vi "_Update TIC Property.vi"(10 "Current Data":T2={"Scan#"=0, "Run Time (mS)"=0, "TIC X"=[], "TIC Y"=[], "MassRange"=[], "Fixed Mass (amu)"=1.0, "Method"={"StartT(mS)"=0, "#Cycles"=0, "PauseT(uS)"=0, "ScanType"=0, "Polarity"=0, "FixedMass"=0.0, "DelayT(mS)"=0, "Active Ch"=[], "Mass Range"=[]}} {"Method"."Mass Range"."Res" items=["High/High", "Medium/Medium", "Low/Low", "High/Medium", "High/Low", "Medium/High", "Medium/Low", "Low/High", "Low/Medium"]}) -> (0 "Run Mode":T1, 1 "YMax":dbl, 2 "TIC Data":cluster{"TIC X":dbl[], "Data in cps":dbl[]}[](array[cluster]), 3 "YTitle":string, 4 "Q2DC Pol":bool, 5 "Q1DC Pol":bool, 6 "MCA":bool, 7 "XTitle":string)   [LabVIEW 2015]
uses:
  Type/_Current Data.ctl
  Type/_XML Expt.ctl
  Type/_XML Lens.ctl
  Type/_Mass Range Property.ctl
  Type/_Mass Range Parameters.ctl
  Type/_RT Res Type.ctl
  Type/_Run Mode.ctl
  Type/_Run Module.ctl
  Configuration/_Global Configuration.vi
panel:
  out "error out":errorcluster
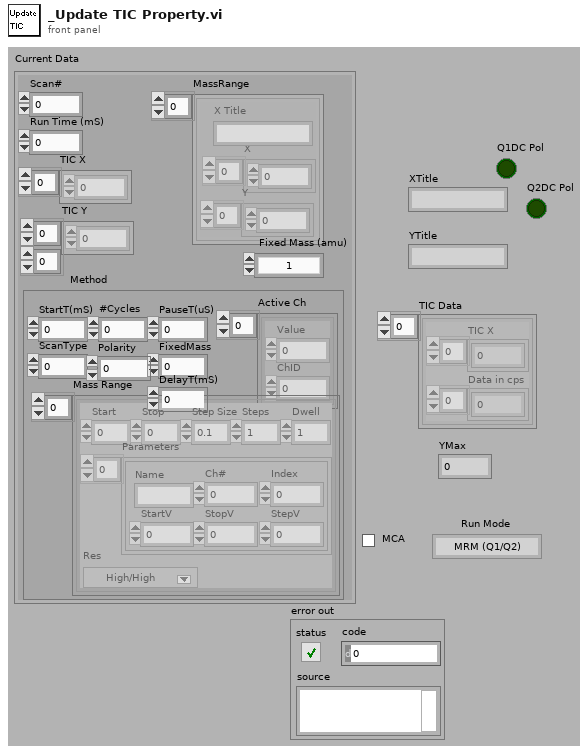
[diagram p1: front panel]
types:
  T1 = typedef "_Run Mode.ctl" = enum16{"MRM (Q1/Q2)", "Q1 Scan", "Q1 SRM", "Q2 Scan", "Q2 SRM", "Product Scan", "Precursor Scan", "Neutral Loss", "Neutral Gain"}
  T2 = typedef "_Current Data.ctl" = cluster{"Scan#":i32, "Run Time (mS)":i32, "TIC X":dbl[], "TIC Y":dbl[][], "MassRange":cluster{"X Title":string, "X":dbl[], "Y":i32[]}[], "Fixed Mass (amu)":dbl, "Method":T3}
  T3 = typedef "_XML Expt.ctl" = cluster{"StartT(mS)":i32, "#Cycles":i32, "PauseT(uS)":i32, "ScanType":i32, "Polarity":u8, "FixedMass":dbl, "DelayT(mS)":i32, "Active Ch":T4[], "Mass Range":T5[]}
  T4 = typedef "_XML Lens.ctl" = cluster{"Value":dbl, "ChID":u8}
  T5 = typedef "_Mass Range Property.ctl" = cluster{"Start":dbl, "Stop":dbl, "Step Size":dbl, "Steps":i32, "Dwell":dbl, "Parameters":T6[], "Res":T7}
  T6 = typedef "_Mass Range Parameters.ctl" = cluster{"Name":string, "Ch#":u8, "StartV":dbl, "StopV":dbl, "StepV":dbl, "Index":u8}
  T7 = typedef "_RT Res Type.ctl" = u16
  T8 = typedef "_Run Module.ctl" = u16
  T9 = typedef "_Lens Property.ctl" = cluster{"Scan Type":u8, "Scans":i32, "Time 1":dbl, "Time 2":dbl, "Value 1":dbl, "Value 2":dbl, "Step Size":dbl}
  T10 = cluster{"Lenses":T9[], "Mass Ranges":T5[], "Acquire":bool, "MCA":bool, "Q1DC EN":bool, "Q1 POL":bool, "Q3 POL":bool, "Q1 RF  EN":bool, "Averaging":bool, "Log Scale":bool, "CPS":bool, "Unit":bool, "Data Path":path, "Run Mode":T1, "Fixed Mass (amu)":dbl, "Q3DC EN":bool, "Q3 RF  EN":bool, "Negative":bool}
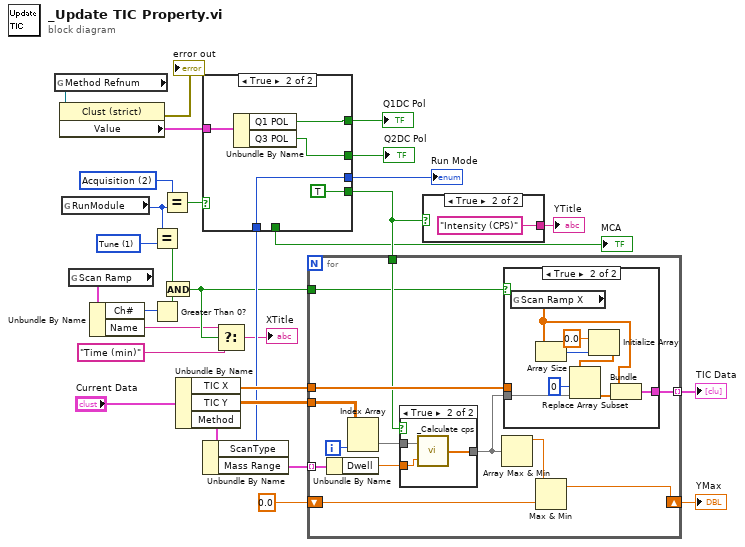
[diagram p0: block diagram]
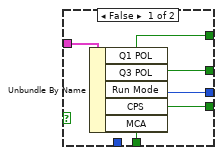
[diagram p2: hidden frame]
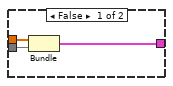
[diagram p3: hidden frame]
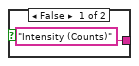
[diagram p5: hidden frame]
diagram:
  w14 = T8 1 items=["Diagnostics", "Tune", "Acquisition"] ("y")
  w16 = T8 2 items=["Diagnostics", "Tune", "Acquisition"] ("y")
  n1 = global read "_Global Configuration.vi" "Method Refnum"() -> (w5:refnum<vi>)
  n2 = property class="Clust (strict)"(reference=w5) -> (error out=→"error out":errorcluster, "Value"=w4:T10)  [unwired: 1 in, 1 out]
  n3 = global read "_Global Configuration.vi" "RunModule"() -> (w15:T8)
  n4 = global read "_Global Configuration.vi" "Scan Ramp"() -> (w13:T6)
  n5 = Unbundle By Name(w13) -> ("Ch#"=w12:u8, "Name"=w7:string)
  n6 = Equal?(x=w15, y=w14) -> (x = y?=w11:bool)
  n7 = Greater Than 0?(x=w12) -> (x > 0?=w10:bool)
  n8 = Equal?(x=w16, y=w15) -> (x = y?=w18:bool)
  n9 = And(x=w11, y=w10) -> (x .and. y?=w9:bool)
  n10 = Unbundle By Name("Current Data") -> ("TIC X"=w29:dbl[], "TIC Y"=w28:dbl[][], "Method"=w27:T3)
  n11 = Unbundle By Name(w27) -> ("ScanType"=w17:i32, "Mass Range"=w19:T5[])
  n12 = case shown="True" w18 {
    tunnel: [w36 TRUE ("CPS")] -> w26
    tunnel: [w35 w41] -> w21
    tunnel: [w34 _] -> w20
    tunnel: w17 -> [_ w41]
    tunnel: w4 -> [w33 w39]
    tunnel: [w32 w38] -> w3
    tunnel: [w31 w37] -> w2
    frame False {
      n13 = Unbundle By Name(w33) -> ("Q1 POL"=w32:bool, "Q3 POL"=w31:bool, "Run Mode"=w35:T1, "CPS"=w36:bool, "MCA"=w34:bool)
    }
    frame True {
      n14 = Unbundle By Name(w39) -> ("Q1 POL"=w38:bool, "Q3 POL"=w37:bool)
    }
  }
  "Run Mode" <- w21
  "MCA" <- w20
  "Q1DC Pol" <- w3
  "Q2DC Pol" <- w2
  n15 = Select(t=w7, s=w9, f="Time (min)") -> (s? t:f=→"XTitle":string)
  n16 = for {
    tunnel: w29 -> [w54]
    tunnel: w28 -> [w53]
    tunnel: [w51] -> w23 mode=indexing
    tunnel: w19 -> [w50] mode=indexing
    tunnel: w26 -> [w49]
    shift-right: [w44] -> w22
    shift-left: 0.0 -> [w46]
    tunnel: w9 -> [w42]
    i -> [w52]
    n17 = Unbundle By Name(w50) -> ("Dwell"=w48:dbl)
    n18 = Index Array(array=w53, index (col)=w52) -> (element=w43:dbl[])  [unwired: 1 in]
    n19 = case shown="True" w49 {
      tunnel: w43 -> [w66 w69]
      tunnel: w48 -> [_ w68]
      tunnel: [w66 w67] -> w47
      frame False {
      }
      frame True {
        n20 = call "_Calculate cps.vi"("Dwell (mS)"=w68, "Raw Counts"=w69) -> ("Data in cps"=w67:dbl[])
      }
    }
    n21 = Array Max & Min(array=w47) -> (max value=w45:dbl)  [unwired: 3 out]
    n22 = case shown="True" w42 {
      tunnel: w54 -> [w57 _]
      tunnel: [w56 w58] -> w51
      tunnel: w47 -> [w55 w61]
      frame False {
        n23 = Bundle("TIC X"=w57, "Data in cps"=w55) -> (w56:cluster{"TIC X":dbl[], "Data in cps":dbl[]})  [unwired: 1 out]
      }
      frame True {
        n24 = global read "_Global Configuration.vi" "Scan Ramp X"() -> (w59:dbl[])
        n25 = Array Size(array=w59) -> (size(s)=w64:i32)
        n26 = Initialize Array(0.0 ("element"), w64) -> (w63:dbl[])
        n27 = Replace Array Subset(array=w63, new element=w61, index=0) -> (w60:dbl[])
        n28 = Bundle("Scan Ramp X"=w59, w60) -> (w58:cluster{"Scan Ramp X":dbl[], dbl[]})  [unwired: 1 out]
      }
    }
    n29 = Max & Min(x=w45, y=w46) -> (max(x,y)=w44:dbl)  [unwired: 1 out]
  }
  "TIC Data" <- w23
  "YMax" <- w22
  n30 = case shown="True" w26 {
    tunnel: ["Intensity (Counts)" "Intensity (CPS)"] -> w24
    frame False {
    }
    frame True {
    }
  }
  "YTitle" <- w24
